vi "Send User Shortcut Menu Selection.vi"(0 "Message Enqueuer in":refnum<class "Message Enqueuer.lvclass">, 5 "CtlRef":refnum<vi>, 7 "Time":u32, 9 "Item Tag":string, 11 "Item Path":string, 12 "Coords":T1, 13 "SubObj":refnum<vi>) -> (15 "error out":errorcluster)   [LabVIEW 2015, in "ActorEvents.lvlib" / "UserShortcutMenuSelectionMsg.lvclass"]
doc: "<License>\nCopyright © 2017 Composed Systems, LLC | All rights reserved\nwww.composed.io\n\nAuthor: Ethan Stern <ethan.stern@composed.io>\n\nThis software is provided \"AS IS\" WITHOUT WARRANTIES, either express or implied, AND IS FOR EDUCATIONAL PURPOSES ONLY.\n</License>"
uses:
  UserShortcutMenuSelectionMsg.lvclass
  <vilib>/ActorFramework/Message Enqueuer/Message Enqueuer.lvclass
  <vilib>/Utility/miscctls.llb/LVPoint32TypeDef.ctl
  UserShortcutMenuSelectionMsg.lvclass/UserShortcutMenuSelectionMsg.ctl
  <vilib>/ActorFramework/Message Enqueuer/Message Enqueuer.lvclass/Message Enqueuer.ctl
  <vilib>/ActorFramework/Message Enqueuer/Enqueue.vi
  <vilib>/ActorFramework/Message Priority Queue/Priority Enqueue.vi
  EventDataMessage/EventDataMessage.lvclass
panel:
  in  "error in (no error)":errorcluster
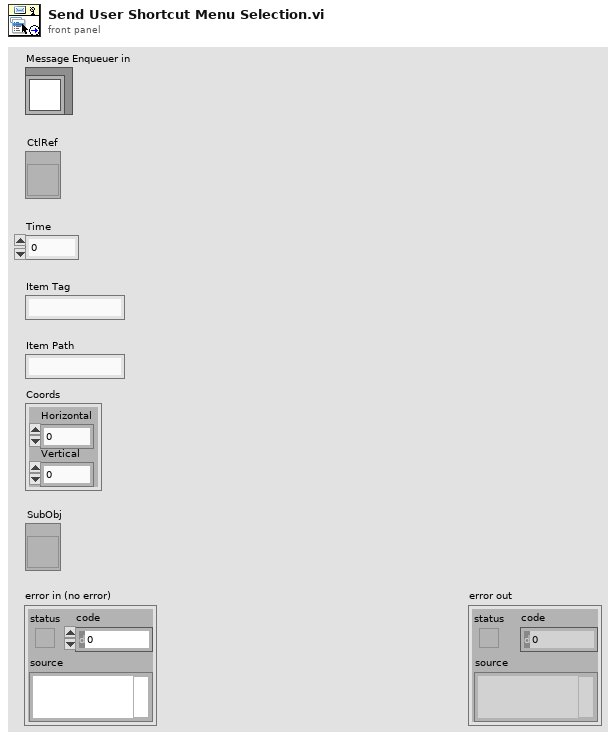
[diagram p1: front panel]
types:
  T1 = typedef "LVPoint32TypeDef.ctl" = cluster{"Horizontal":i32, "Vertical":i32}
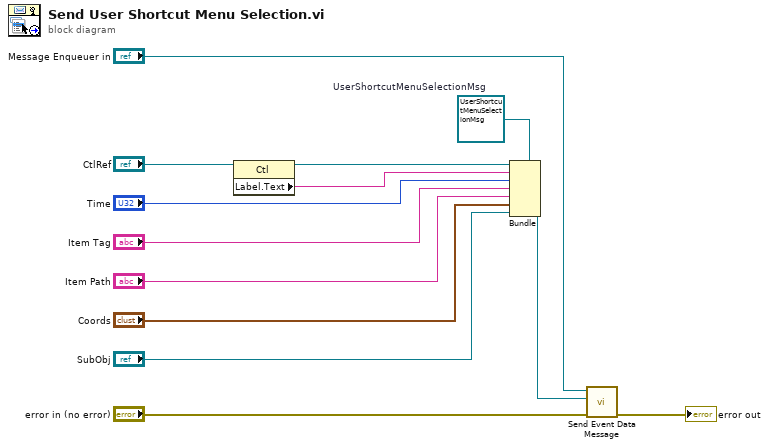
[diagram p0: block diagram]
diagram:
  w13 = refnum<class "UserShortcutMenuSelectionMsg.lvclass"> refnum  # UserShortcutMenuSelectionMsg
  n1 = property class="Ctl"(reference="CtlRef") -> (reference out=w7:refnum<vi>, "Label.Text"=w1:string)  [unwired: 1 in, 1 out]
  n2 = Bundle(cluster=w13, w7, w1, "Time", "Item Tag", "Item Path", "Coords", "SubObj") -> (w10:refnum<class "UserShortcutMenuSelectionMsg.lvclass">)
  n3 = call "Send Event Data Message.vi"("error in (no error)"="error in (no error)", "EventDataMessage in"=w10, "Message Enqueuer in"="Message Enqueuer in") -> ("error out"=→"error out":errorcluster)  [unwired: 8 in]
